vi "Query OPC Bool.vi"(8 "error in (no error)":errorcluster, 9 "NodeID In":string, 10 "Parent NodeID In":string, 11 "OPC UA client refnum in":T1) -> (0 "error out":errorcluster, 1 "Found Out":bool, 2 "Boolean Out":bool, 3 "OPC UA client refnum out":T1)   [LabVIEW 2024, in "OPCUA.lvlib"]
uses:
  <vilib>/OPCUA/controls/OPC UA Client Refnum.ctl
  OPCUA.lvlib
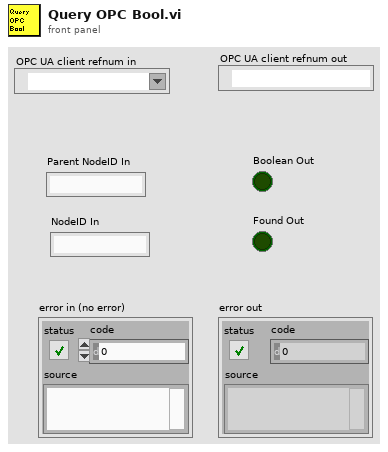
[diagram p1: front panel]
types:
  T1 = typedef "OPC UA Client Refnum.ctl" = refnum<k21>
  T2 = typedef "Read Variant Result.ctl" = cluster{"node ID":T3, "value ":variant, "timestamp":timestamp, "status":T4}
  T3 = typedef "NodeId.ctl" = string
  T4 = typedef "OPC UA StatusCode.ctl" = u32
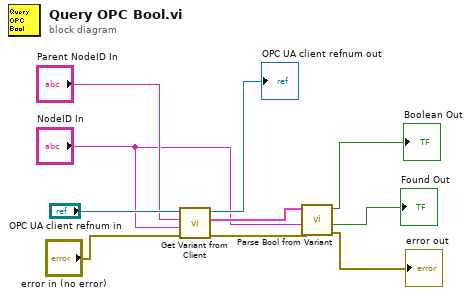
[diagram p0: block diagram]
diagram:
  n1 = call "Get Variant from Client.vi"("error in (no error)"="error in (no error)", "NodeID In"="NodeID In", "Parent NodeID In"="Parent NodeID In", "OPC UA client refnum in"="OPC UA client refnum in") -> ("error out"=w5:errorcluster, "Variant results out"=w6:T2[], "OPC UA client refnum out"=→"OPC UA client refnum out":T1)  [unwired: 5 in]
  n2 = call "Parse Bool from Variant.vi"("error in (no error)"=w5, "Node ID In"="NodeID In", "Variant results In"=w6) -> ("error out"=→"error out":errorcluster, "Result Found?"=→"Found Out":bool, "Boolean Out"=→"Boolean Out":bool)  [unwired: 6 in]
